vi "niScope Export Signal.vi"(0 "instrument handle":refnum<k15>, 1 "signal identifier":T1="None" caption="signal identifier (None)", 5 "signal":T3=2 caption="signal (Start Trigger)" items=["Start Trigger"=2, "Advance Trigger"=5, "Reference Trigger"=1, "End of Record Event"=4, "End of Acquisition Event"=3, "Ready for Start Event"=7, "Ready for Advance Event"=6, "Ready for Reference Event"=10, "Reference Clock"=100, "Sample Clock"=101, "5 Volt Power"=13], 9 "output terminal":T2="VAL_NO_SOURCE" caption="output terminal (None)", 11 "error in":errorcluster) -> (4 "instrument handle out":refnum<k15>, 15 "error out":errorcluster)   [LabVIEW 2013]
doc: "Configures the digitizer to generate a signal that other devices can detect when configured for digital triggering or sharing clocks. The <B>signal</B> parameter specifies what condition causes the digitizer to generate the signal. The <B>output terminal</B> parameter specifies where to send the signal on the hardware (such as a PFI connector or RTSI line)."
uses:
  <instrlib>/niScope/Controls/niScope exportable signals.ctl
  <instrlib>/niScope/Controls/niScope export destinations.ctl
  <instrlib>/niScope/Controls/niScope which signal.ctl
  niScope_32.dll
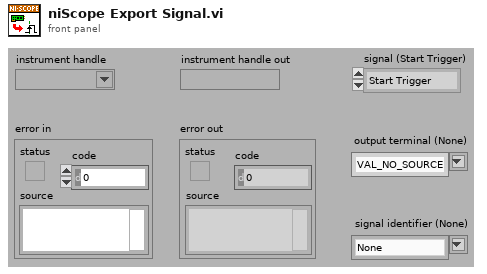
[diagram p1: front panel]
types:
  T1 = typedef "niScope which signal.ctl" = string
  T2 = typedef "niScope export destinations.ctl" = string
  T3 = typedef "niScope exportable signals.ctl" = u16
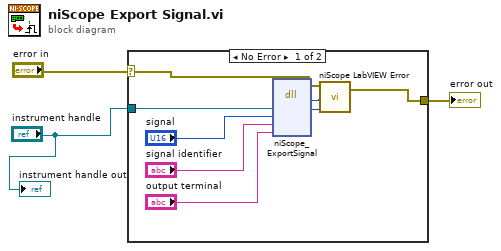
[diagram p0: block diagram]
diagram:
  n1 = case shown="No Error" "error in" {
    selector: "error in" -> [w6 w12]
    tunnel: [w7 w12] -> w3
    tunnel: "instrument handle" -> [w11 _]
    frame No Error {
      n2 = dll-call lib="niScope_*.*" fn="niScope_ExportSignal"("instrument handle"=w11, "signal"="signal", "signalIdentifier"="signal identifier", "outputTerminal"="output terminal") -> ("status"=w8:i32, "instrument handle"=w9:u32)  [unwired: 6 in, 2 out]
      n3 = call <instrlib>:"niScope LabVIEW Error.vi"("instrument handle"=w9, "niScope error code (0)"=w8, "error in (no error)"=w6) -> ("error out"=w7:errorcluster)  [unwired: 2 in]
    }
    frame Error {
    }
  }
  "error out" <- w3
  "instrument handle out" <- "instrument handle"
